vi "ExProg_Tick.vi"(0 "Simulation?":bool, 5 "Timestep (s)":dbl, 9 "Program":T8, 11 "Current time (s)":dbl, 12 "Script exec state in":T7) -> (3 "Script exec state out":T7, 6 "Instruction index":i32, 8 "Last instruction":T4={"cmd"=enum."wait", "axis"=enum."magrot", "value/pos"=0.0, "speed"=0.0, "name"=""}, 10 "script ended?":bool, 14 "Last command":T5)   [LabVIEW 2011]
uses:
  ExperimentProgramType.ctl
  ExProgCommandType.ctl
  ExProgCommandEnumType.ctl
  Motors/MotorAxisEnum.ctl
  Motors/MotorPosType.ctl
  Typedefs/XYf.ctl
  Motors/MotorPosFlagsType.ctl
  ExProgState.ctl
  ScriptEventType.ctl
panel:
  out "Motor Axis accuracy conditions":T1
  out "Axis flags":T3
  # "(used for commands with string parameters)"
  # "(used for commands with string parameters)"
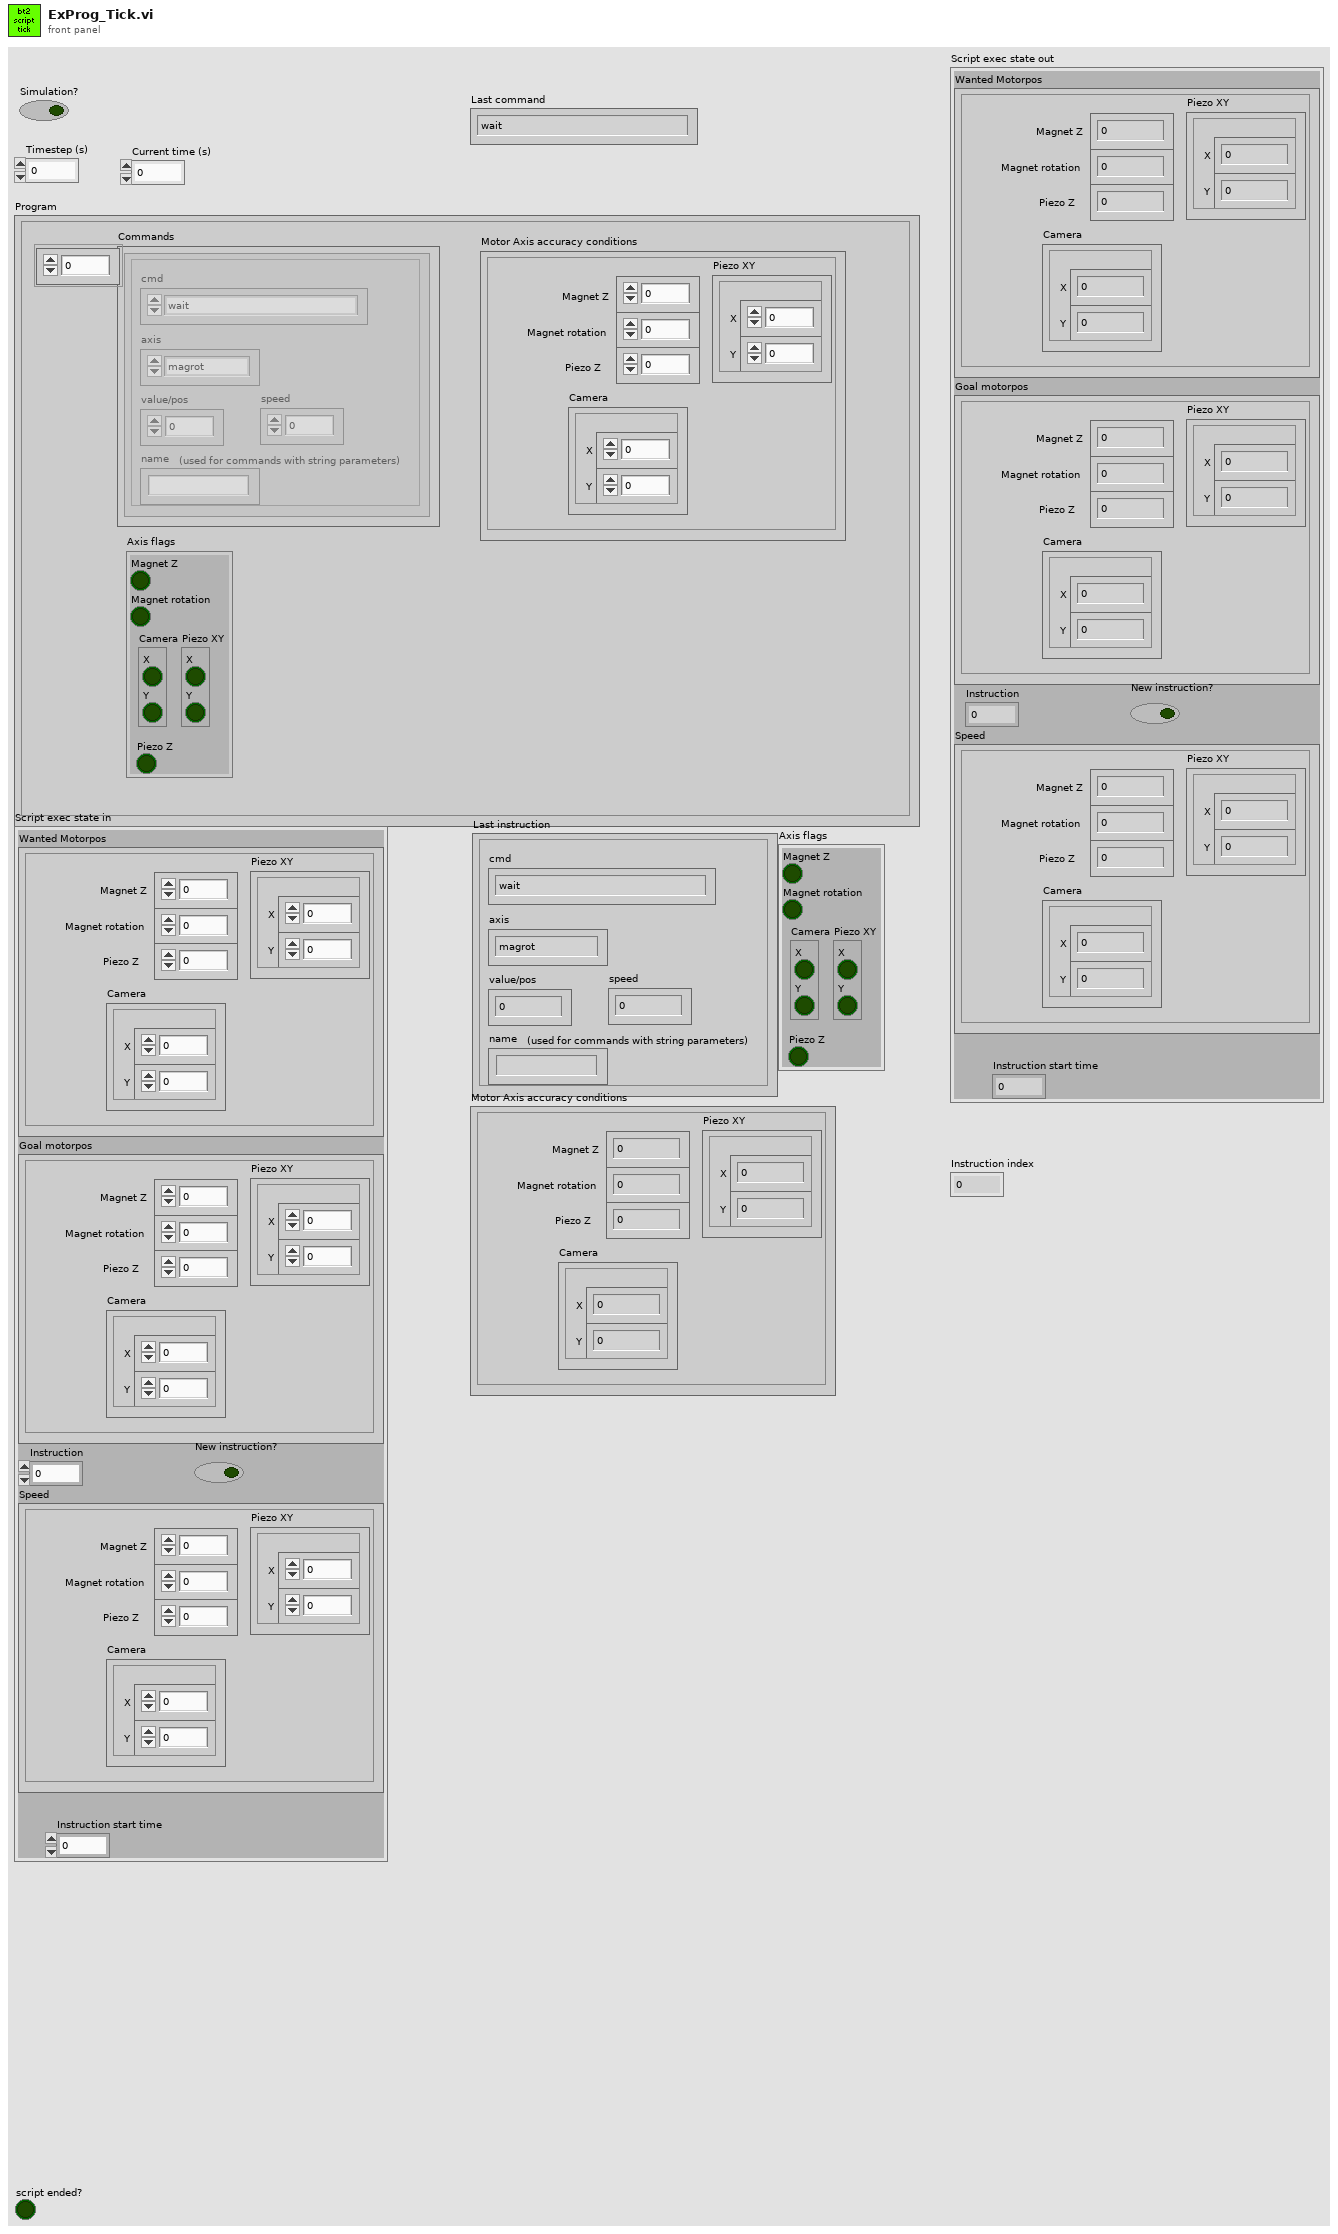
[diagram p1: front panel]
types:
  T1 = typedef "MotorPosType.ctl" = cluster{"Magnet Z":dbl, "Magnet rotation":dbl, "Camera":T2, "Piezo XY":T2, "Piezo Z":dbl}
  T2 = typedef "XYf.ctl" = cluster{"X":sgl, "Y":sgl}
  T3 = typedef "MotorPosFlagsType.ctl" = cluster{"Magnet Z":bool, "Magnet rotation":bool, "Camera":cluster{"X":bool, "Y":bool}, "Piezo XY":cluster{"X":bool, "Y":bool}, "Piezo Z":bool}
  T4 = typedef "ExProgCommandType.ctl" = cluster{"cmd":T5, "axis":T6, "value/pos":dbl, "speed":dbl, "name":string}
  T5 = typedef "ExProgCommandEnumType.ctl" = enum16{"wait", "move", "event", "idle", "when", "section", "stop"}
  T6 = typedef "MotorAxisEnum.ctl" = enum16{"no axis", "magrot", "magpos", "px", "py", "pz", "camx", "camy"}
  T7 = typedef "ExProgState.ctl" = cluster{"Wanted Motorpos":T1, "Goal motorpos":T1, "Instruction":i32, "Speed":T1, "New instruction?":bool, "Instruction start time":dbl}
  T8 = typedef "ExperimentProgramType.ctl" = cluster{"Commands":T4[], "Motor Axis accuracy conditions":T1, "Axis flags":T3}
  T9 = typedef "ScriptEventType.ctl" = cluster{"Text":string}
  T10 = cluster{"Magnet Z":i16, "Magnet rotation":i16, "Camera":cluster{"X":i16, "Y":i16}, "Piezo XY":cluster{"X":i16, "Y":i16}, "Piezo Z":i16}
  T11 = typedef "QueueListType.ctl" = cluster{"Motor In":refnum<queue>, "User Interface Image View":refnum<queue>, "User Interface Camera Control":refnum<queue>, "User Interface Event Notifier":refnum<notifier>, "Initialized?":bool, "Experiment Script Event Notifier":refnum<notifier>}
  T12 = cluster{"Magnet Z":dbl, "Magnet rotation":dbl, "Camera":cluster{"X":dbl, "Y":dbl}, "Piezo XY":cluster{"X":dbl, "Y":dbl}, "Piezo Z":dbl}
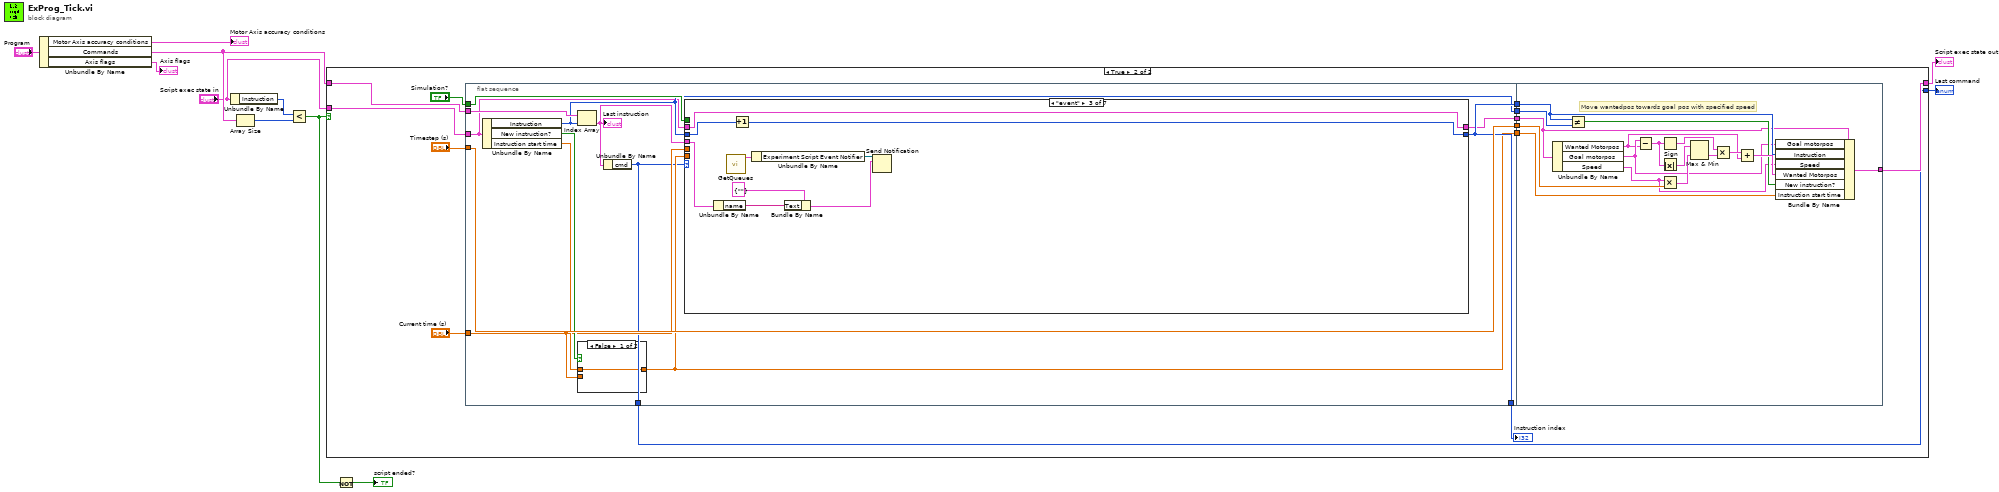
[diagram p0: block diagram]
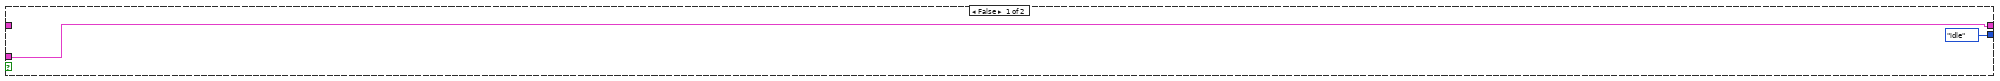
[diagram p2: hidden frame]
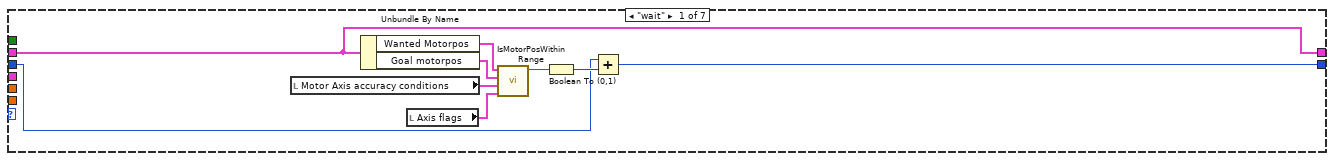
[diagram p4: hidden frame]
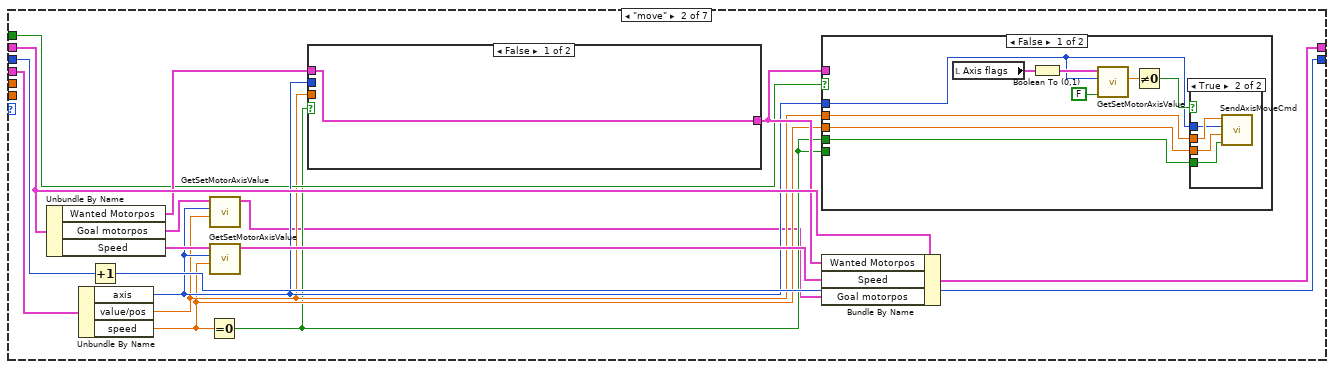
[diagram p5: hidden frame]
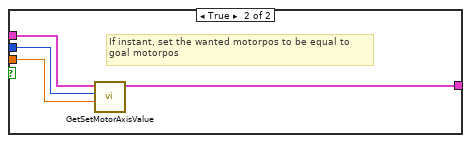
[diagram p8: hidden frame]
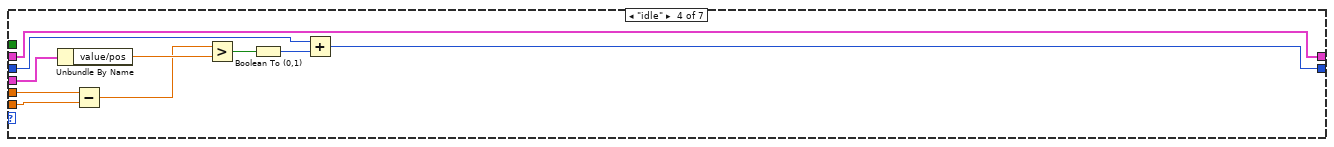
[diagram p9: hidden frame]
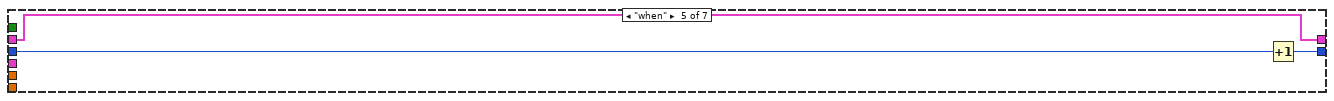
[diagram p10: hidden frame]
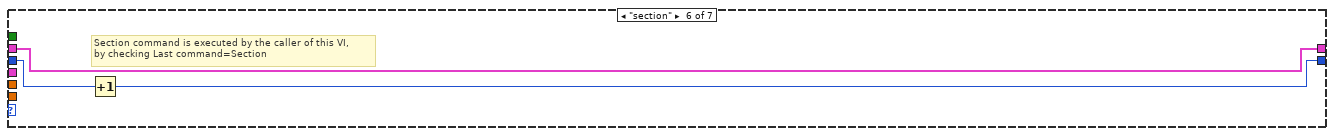
[diagram p11: hidden frame]
diagram:
  n1 = Unbundle By Name("Program") -> ("Motor Axis accuracy conditions"=→"Motor Axis accuracy conditions":T1, "Commands"=w9:T4[], "Axis flags"=→"Axis flags":T3)
  n2 = Unbundle By Name("Script exec state in") -> ("Instruction"=w7:i32)
  n3 = Array Size(array=w9) -> (size(s)=w6:i32)
  n4 = Less?(x=w7, y=w6) -> (x < y?=w4:bool)
  n5 = case shown="True" w4 {
    tunnel: "Script exec state in" -> [w13 w23]
    tunnel: w9 -> [_ w19]
    tunnel: [w13 w18] -> w2
    tunnel: [ExProgCommandEnumType."idle" ("cmd") w14] -> w1
    frame False {
    }
    frame True {
      n6 = flat-sequence {
        tunnel: "Timestep (s)" -> [w39]
        tunnel: "Simulation?" -> [w37]
        tunnel: [w39] -> w26
        tunnel: [w35] -> w21
        tunnel: w23 -> [w28]
        tunnel: [w27] -> w25
        tunnel: [w35] -> w24
        tunnel: w19 -> [w36]
        tunnel: "Current time (s)" -> [w31]
        tunnel: [w34] -> w16
        tunnel: [w30] -> w15
        tunnel: [w29] -> w14
        tunnel: w26 -> [w122]
        tunnel: w25 -> [w115]
        tunnel: w24 -> [w118]
        tunnel: [w121] -> w18
        tunnel: w16 -> [w117]
        tunnel: w15 -> [w119]
        frame #0 {
          n7 = Unbundle By Name(w28) -> ("Instruction"=w34:i32, "New instruction?"=w33:bool, "Instruction start time"=w32:dbl)
          n8 = Index Array(array=w36, index=w34) -> (element=w38:T4)
          "Last instruction" <- w38
          n9 = case shown="False" w33 {
            tunnel: [w40 w41] -> w30
            tunnel: w32 -> [w40 _]
            tunnel: w31 -> [_ w41]
            frame False {
            }
            frame True {
            }
          }
          n10 = Unbundle By Name(w38) -> ("cmd"=w29:T5)
          n11 = case shown="\"event\"" w29 {
            tunnel: w34 -> [w49 w66 w93 w98 w106 w109 w111]
            tunnel: [w48 w65 w92 w95 w105 w108 w111] -> w35
            tunnel: w38 -> [_ w64 w91 w102 _ _ _]
            tunnel: w37 -> [_ w55 _ _ _ _ _]
            tunnel: w31 -> [_ _ _ w103 _ _ _]
            tunnel: w30 -> [_ _ _ w100 _ _ _]
            tunnel: [w42 w62 w90 w94 w104 w107 w110] -> w27
            tunnel: w28 -> [w42 w63 w90 w94 w104 w107 w110]
            frame "wait" {
              n12 = local read "Motor Axis accuracy conditions"() -> (w43:T1)
              n13 = Unbundle By Name(w42) -> ("Wanted Motorpos"=w46:T1, "Goal motorpos"=w45:T1)
              n14 = local read "Axis flags"() -> (w44:T3)
              n15 = call "IsMotorPosWithinRange.vi"("Which axis?"=w44, "Allowed difference"=w43, "Wanted Position"=w45, "Current Position"=w46) -> ("In range?"=w47:bool)  [unwired: 7 in]
              n16 = Boolean To (0,1)(Boolean=w47) -> (0, 1=w50:i16)
              n17 = Add(x=w49, y=w50) -> (x+y=w48:i32)
            }
            frame "move" {
              n18 = Unbundle By Name(w63) -> ("Wanted Motorpos"=w58:T1, "Goal motorpos"=w59:T1, "Speed"=w61:T1)
              n19 = Unbundle By Name(w64) -> ("axis"=w56:T6, "value/pos"=w54:dbl, "speed"=w53:dbl)
              n20 = Increment(x=w66) -> (x+1=w65:i32)
              n21 = Equal To 0?(x=w53) -> (x = 0?=w52:bool)
              n22 = call "GetSetMotorAxisValue.vi"("pos"=w54, "axis"=w56, "Motorpos in"=w59) -> ("Motorpos out"=w51:T1)  [unwired: 7 in, 1 out]
              n23 = call "GetSetMotorAxisValue.vi"("pos"=w53, "axis"=w56, "Motorpos in"=w61) -> ("Motorpos out"=w60:T1)  [unwired: 7 in, 1 out]
              n24 = case shown="False" w52 {
                tunnel: w56 -> [_ w84]
                tunnel: w54 -> [_ w83]
                tunnel: w58 -> [w80 w82]
                tunnel: [w80 w81] -> w57
                frame False {
                }
                frame True {
                  # "If instant, set the wanted motorpos to be equal to \ngoal motorpos"
                  n25 = call "GetSetMotorAxisValue.vi"("pos"=w83, "axis"=w84, "Motorpos in"=w82) -> ("Motorpos out"=w81:T1)  [unwired: 7 in, 1 out]
                }
              }
              n26 = case shown="False" w55 {
                tunnel: w57 -> [_ _]
                tunnel: w52 -> [_ _]
                tunnel: w56 -> [w69 _]
                tunnel: w54 -> [w70 _]
                tunnel: w53 -> [w68 _]
                tunnel: w52 -> [w67 _]
                frame False {
                  n27 = local read "Axis flags"() -> (w75:T3)
                  n28 = Boolean To (0,1)(Boolean=w75) -> (0, 1=w74:T10)
                  n29 = call "GetSetMotorAxisValue.vi"("set? (T)"=FALSE, "axis"=w69, "Motorpos in"=w74) -> ("pos (out)"=w72:dbl)  [unwired: 7 in, 1 out]
                  n30 = Not Equal To 0?(x=w72) -> (x != 0?=w71:bool)
                  n31 = case shown="True" w71 {
                    tunnel: w70 -> [_ w79]
                    tunnel: w69 -> [_ w78]
                    tunnel: w68 -> [_ w77]
                    tunnel: w67 -> [_ w76]
                    frame False {
                    }
                    frame True {
                      n32 = call "SendAxisMoveCmd.vi"("Instant? (T)"=w76, "Speed"=w77, "axis"=w78, "Position"=w79) -> ()  [unwired: 7 in, 1 out]
                    }
                  }
                }
                frame True {
                }
              }
              n33 = Bundle By Name(cluster=w63, "Wanted Motorpos"=w57, "Speed"=w60, "Goal motorpos"=w51) -> (w62:T7)
            }
            frame "event" {
              n34 = Unbundle By Name(w91) -> ("name"=w85:string)
              n35 = call "GetQueues.vi"() -> ("Queue List"=w89:T11)  [unwired: 10 in, 1 out]
              n36 = Increment(x=w93) -> (x+1=w92:i32)
              n37 = Unbundle By Name(w89) -> ("Experiment Script Event Notifier"=w88:refnum<notifier>)
              n38 = Bundle By Name(cluster=T9 {"Text"=""} ("notification"), "Text"=w85) -> (w86:T9)
              n39 = Send Notification(notification=w86, notifier=w88) -> ()  [unwired: 1 in, 2 out]
            }
            frame "idle" {
              n40 = Unbundle By Name(w102) -> ("value/pos"=w101:dbl)
              n41 = Subtract(x=w103, y=w100) -> (x-y=w99:dbl)
              n42 = Greater?(x=w99, y=w101) -> (0:w96:bool)
              n43 = Boolean To (0,1)(Boolean=w96) -> (0, 1=w97:i16)
              n44 = Add(x=w98, y=w97) -> (x+y=w95:i32)
            }
            frame "when" {
              n45 = Increment(x=w106) -> (x+1=w105:i32)
            }
            frame "section" {
              # "Section command is executed by the caller of this VI, \nby checking Last command=Section"
              n46 = Increment(x=w109) -> (x+1=w108:i32)
            }
            frame "stop", Default {
              # "Stop command is implemented in caller by checking for Last command=stop"
            }
          }
        }
        frame #1 {
          # "Move wantedpos towards goal pos with specified speed"
          n47 = Unbundle By Name(w115) -> ("Wanted Motorpos"=w113:T1, "Goal motorpos"=w114:T1, "Speed"=w112:T1)
          n48 = Not Equal?(x=w118, y=w117) -> (x != y?=w116:bool)
          n49 = Subtract(x=w114, y=w113) -> (x-y=w127:T1)
          n50 = Sign(1:w127) -> (0:w125:T1)
          n51 = Absolute Value(x=w127) -> (abs(x)=w128:T1)
          n52 = Multiply(x=w112, y=w122) -> (x*y=w124:T12)
          n53 = Max & Min(x=w128, y=w124) -> (min(x,y)=w126:T12)  [unwired: 1 out]
          n54 = Multiply(x=w125, y=w126) -> (x*y=w123:T12)
          n55 = Add(x=w123, y=w113) -> (x+y=w120:T12)
          n56 = Bundle By Name(cluster=w115, "Goal motorpos"=w114, "Instruction"=w118, "Speed"=w112, "Wanted Motorpos"=w120, "New instruction?"=w116, "Instruction start time"=w119) -> (w121:T7)
        }
      }
      "Instruction index" <- w21
    }
  }
  "Script exec state out" <- w2
  "Last command" <- w1
  n57 = Not(x=w4) -> (.not. x?=→"script ended?":bool)
